vi "Rig_Pict_Display_Pref.vi"(0 "Traverse Name":string) -> (1 "Co-ordinate Transform":bool, 4 "Which Axis is vertical?":enum16{"X Axis", "Y Axis", "Z Axis"}(ring), 6 "Plan View":T1, 7 "Side View":T1, 8 "Front View":T1)   [LabVIEW 2010]
uses:
  Pict_Plot_Axis.ctl
  Axis.ctl
  Globals/Constants_global.vi
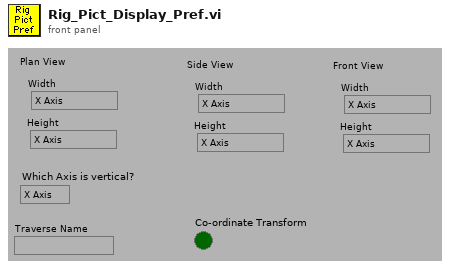
[diagram p1: front panel]
types:
  T1 = typedef "Pict_Plot_Axis.ctl" = cluster{"Width":T2, "Height":T2}
  T2 = typedef "Axis.ctl" = enum16{"X Axis", "X Axis -ve", "Y Axis", "Y Axis -ve", "Z Axis", "Z Axis -ve"}
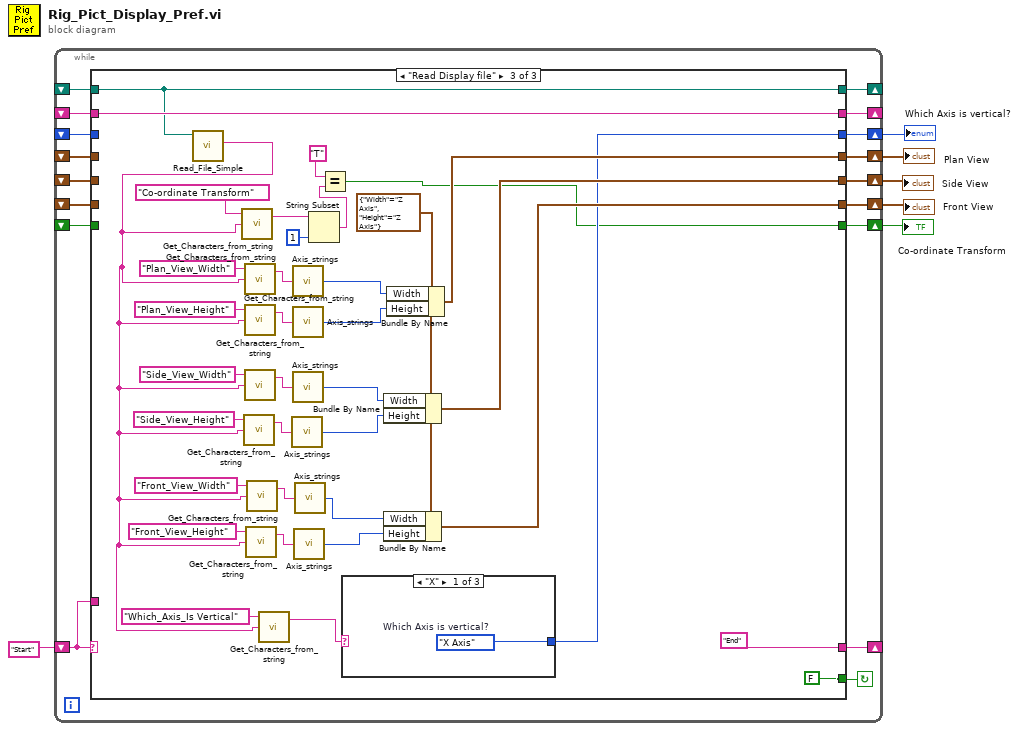
[diagram p0: block diagram]
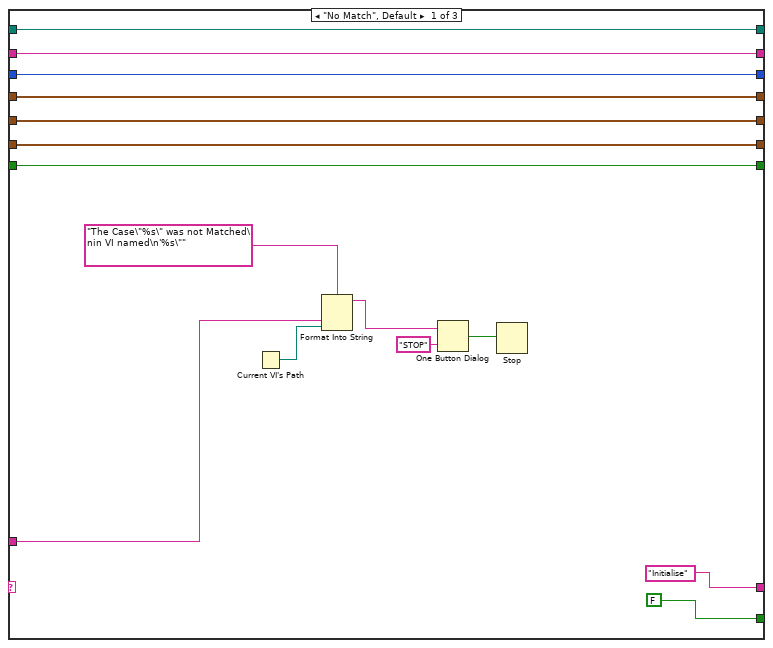
[diagram p2: hidden frame]
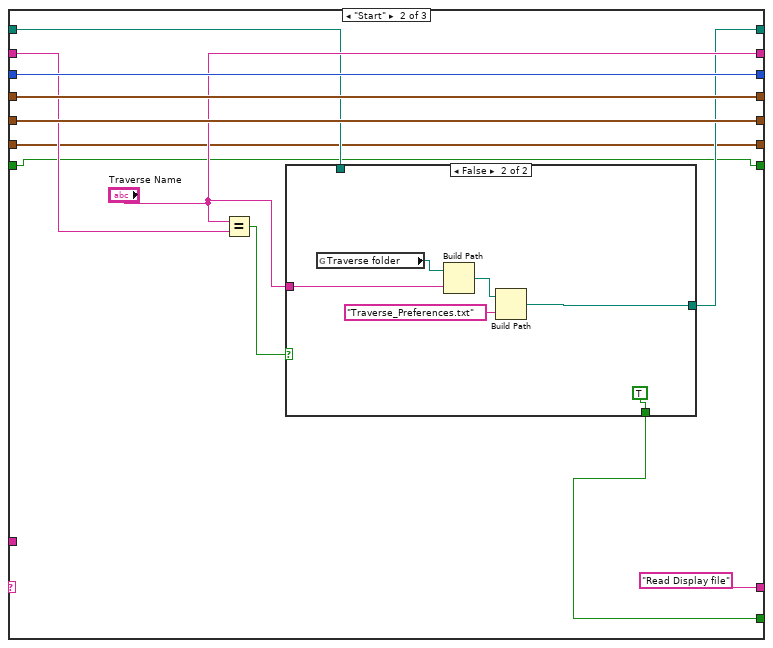
[diagram p3: hidden frame]
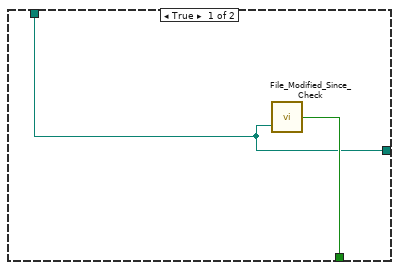
[diagram p4: hidden frame]
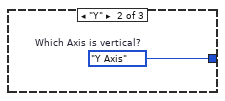
[diagram p5: hidden frame]
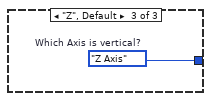
[diagram p6: hidden frame]
diagram:
  n1 = while {
    shift-left: "Start" -> [w21]
    shift-right: [w22] -> _
    shift-right: [w19] -> _
    shift-left: _ -> [w20]
    shift-right: [w13] -> w2
    shift-left: _ -> [w14]
    shift-right: [w16] -> w5
    shift-left: _ -> [w15]
    shift-right: [w17] -> w4
    shift-left: _ -> [w18]
    shift-right: [w12] -> _
    shift-left: _ -> [w11]
    shift-right: [w9] -> w3
    shift-left: _ -> [w10]
    shift-right: [w8] -> w1
    shift-left: _ -> [w7]
    stop <- w23 continue-if-true
    n2 = case shown="\"Read Display file\"" w21 {
      tunnel: [FALSE w43 FALSE ("Modified?")] -> w23
      tunnel: ["Initialise" "Read Display file" "End"] -> w22
      tunnel: w21 -> [w33 _ _]
      tunnel: w20 -> [w29 w46 w93]
      tunnel: [w29 "Traverse Name" w93] -> w19
      tunnel: w18 -> [w26 w49 _]
      tunnel: [w26 w49 w71] -> w17
      tunnel: [w27 w48 w72] -> w16
      tunnel: w15 -> [w27 w48 _]
      tunnel: w14 -> [w28 w47 _]
      tunnel: [w28 w47 w67] -> w13
      tunnel: [w30 w44 w92] -> w12
      tunnel: w11 -> [w30 w41 w92]
      tunnel: w10 -> [w25 w40 _]
      tunnel: [w25 w40 w70] -> w9
      tunnel: [w24 w39 w60] -> w8
      tunnel: w7 -> [w24 w39 _]
      frame "No Match", Default {
        n3 = Current VI's Path() -> (path=w32:path)
        n4 = Format Into String(format string="The Case\"%s\" was not Matched\nin VI named\n'%s\"" ("Format String"), w33, w32) -> (resulting string=w36:string)  [unwired: 2 in, 1 out]
        n5 = One Button Dialog(message=w36, button name ("OK")="STOP") -> (true=w34:bool)
        n6 = Stop(stop? (T)=w34) -> ()
      }
      frame "Start" {
        n7 = Equal?(x="Traverse Name", y=w46) -> (x = y?=w42:bool)
        n8 = case shown="False" w42 {
          tunnel: "Traverse Name" -> [_ w57]
          tunnel: [w51 w54] -> w44
          tunnel: [w52 TRUE ("Modified?")] -> w43
          tunnel: w41 -> [w51 _]
          frame True {
            n9 = call "File_Modified_Since_Check.vi"("Pathname"=w51) -> ("Modified?"=w52:bool)  [unwired: 1 in]
          }
          frame False {
            n10 = global read "Constants_global.vi" "Traverse folder"() -> (w58:path)
            n11 = Build Path(base path=w58, name or relative path=w57) -> (appended path=w56:path)
            n12 = Build Path(base path=w56, name or relative path="Traverse_Preferences.txt") -> (appended path=w54:path)
          }
        }
      }
      frame "Read Display file" {
        w77 = T1 {"Width"=enum."Z Axis", "Height"=enum."Z Axis"} ("Plot Axis")
        n13 = call "Read_File_Simple.vi"("Filename"=w92) -> ("string"=w59:string)  [unwired: 2 in, 7 out]
        n14 = call "Get_Characters_from_string.vi"("Input string"=w59, "Variable name"="Co-ordinate Transform") -> ("Value"=w63:string)  [unwired: 1 in, 1 out]
        n15 = call "Get_Characters_from_string.vi"("Input string"=w59, "Variable name"="Side_View_Height") -> ("Value"=w85:string)  [unwired: 1 in, 1 out]
        n16 = call "Get_Characters_from_string.vi"("Input string"=w59, "Variable name"="Plan_View_Width") -> ("Value"=w90:string)  [unwired: 1 in, 1 out]
        n17 = call "Get_Characters_from_string.vi"("Input string"=w59, "Variable name"="Plan_View_Height") -> ("Value"=w89:string)  [unwired: 1 in, 1 out]
        n18 = call "Get_Characters_from_string.vi"("Input string"=w59, "Variable name"="Side_View_Width") -> ("Value"=w86:string)  [unwired: 1 in, 1 out]
        n19 = call "Get_Characters_from_string.vi"("Input string"=w59, "Variable name"="Front_View_Height") -> ("Value"=w81:string)  [unwired: 1 in, 1 out]
        n20 = call "Get_Characters_from_string.vi"("Input string"=w59, "Variable name"="Front_View_Width") -> ("Value"=w82:string)  [unwired: 1 in, 1 out]
        n21 = call "Get_Characters_from_string.vi"("Input string"=w59, "Variable name"="Which_Axis_Is Vertical") -> ("Value"=w68:string)  [unwired: 1 in, 1 out]
        n22 = call "Axis_strings.vi"("String"=w85) -> ("Enum"=w73:T2)
        n23 = call "Axis_strings.vi"("String"=w90) -> ("Enum"=w76:T2)
        n24 = call "Axis_strings.vi"("String"=w89) -> ("Enum"=w75:T2)
        n25 = call "Axis_strings.vi"("String"=w86) -> ("Enum"=w74:T2)
        n26 = call "Axis_strings.vi"("String"=w81) -> ("Enum"=w78:T2)
        n27 = call "Axis_strings.vi"("String"=w82) -> ("Enum"=w79:T2)
        n28 = String Subset(string=w63, length (rest)=1 ("length (rest)")) -> (substring=w61:string)  [unwired: 1 out]
        n29 = Equal?(x="T", y=w61) -> (x = y?=w60:bool)
        n30 = case shown="\"X\"" w68 {
          tunnel: [w95 w96 w97] -> w67
          frame "X" {
            w95 = enum16{"X Axis", "Y Axis", "Z Axis"}."X Axis"  # Which Axis is vertical?
          }
          frame "Y" {
            w96 = enum16{"X Axis", "Y Axis", "Z Axis"}."Y Axis"  # Which Axis is vertical?
          }
          frame "Z", Default {
            w97 = enum16{"X Axis", "Y Axis", "Z Axis"}."Z Axis"  # Which Axis is vertical?
          }
        }
        n31 = Bundle By Name(cluster=w77, "Width"=w74, "Height"=w73) -> (w71:T1)
        n32 = Bundle By Name(cluster=w77, "Width"=w79, "Height"=w78) -> (w70:T1)
        n33 = Bundle By Name(cluster=w77, "Width"=w76, "Height"=w75) -> (w72:T1)
      }
    }
  }
  "Plan View" <- w5
  "Side View" <- w4
  "Front View" <- w3
  "Which Axis is vertical?" <- w2
  "Co-ordinate Transform" <- w1
